vi "Get Current Temperature.vi"(8 "error in (no error)":cluster{"状态":bool, "代码":i32, "源":string} caption="错误输入（无错误）", 11 "冷却器输入":refnum<class "Cooler.lvclass">) -> (0 "error out":cluster{"状态":bool, "代码":i32, "源":string} caption="错误输出", 2 "水位":dbl)   [LabVIEW 2013, in "Cooler.lvlib" / "Cooler.lvclass"]
doc: "从传感器或仿真硬件读取当前温度。"
uses:
  Cooler.lvclass
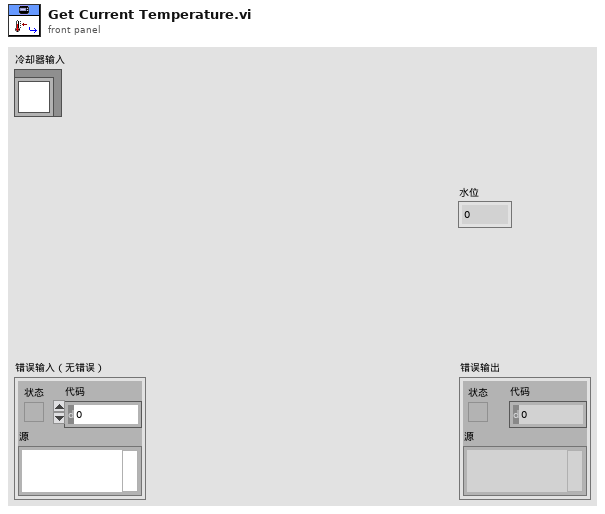
[diagram p1: front panel]
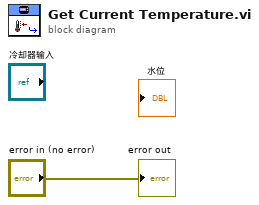
[diagram p0: block diagram]
diagram:
  "error out" <- "error in (no error)"
